vi "All Not Complex.vi"() -> (3 "Benchmark":cluster{i32[], dbl[]}[](graph))   [LabVIEW 2020]
doc: "Execute GEMM Process for different size on different Toolkits (Accelerator/Culab/CUDA/LabVIEW/G2CPU) and LabVIEW(CPU)."
uses:
  Source/_Controls/acc_execution_provider_enum.ctl
panel:
  out "Accelerator CUDA":bool
  out "Culab":bool
  out "Accelerator TRT":bool
  out "LabVIEW":bool
  out "G2CPU":bool
  out "LabVIEW Toolkit Time":dbl
  out "G2CPU Time":dbl
  out "Accelerator CUDA Times":dbl[](array[numeric])
  out "Accelerator CUDA Time":dbl
  out "LabVIEW Times":dbl[](array[numeric])
  out "G2CPU Times":dbl[](array[numeric])
  out "Culab Times":dbl[](array[numeric])
  out "Accelerator TRT Times":dbl[](array[numeric])
  out "Culab Time":dbl
  out "Accelerator TRT Time":dbl
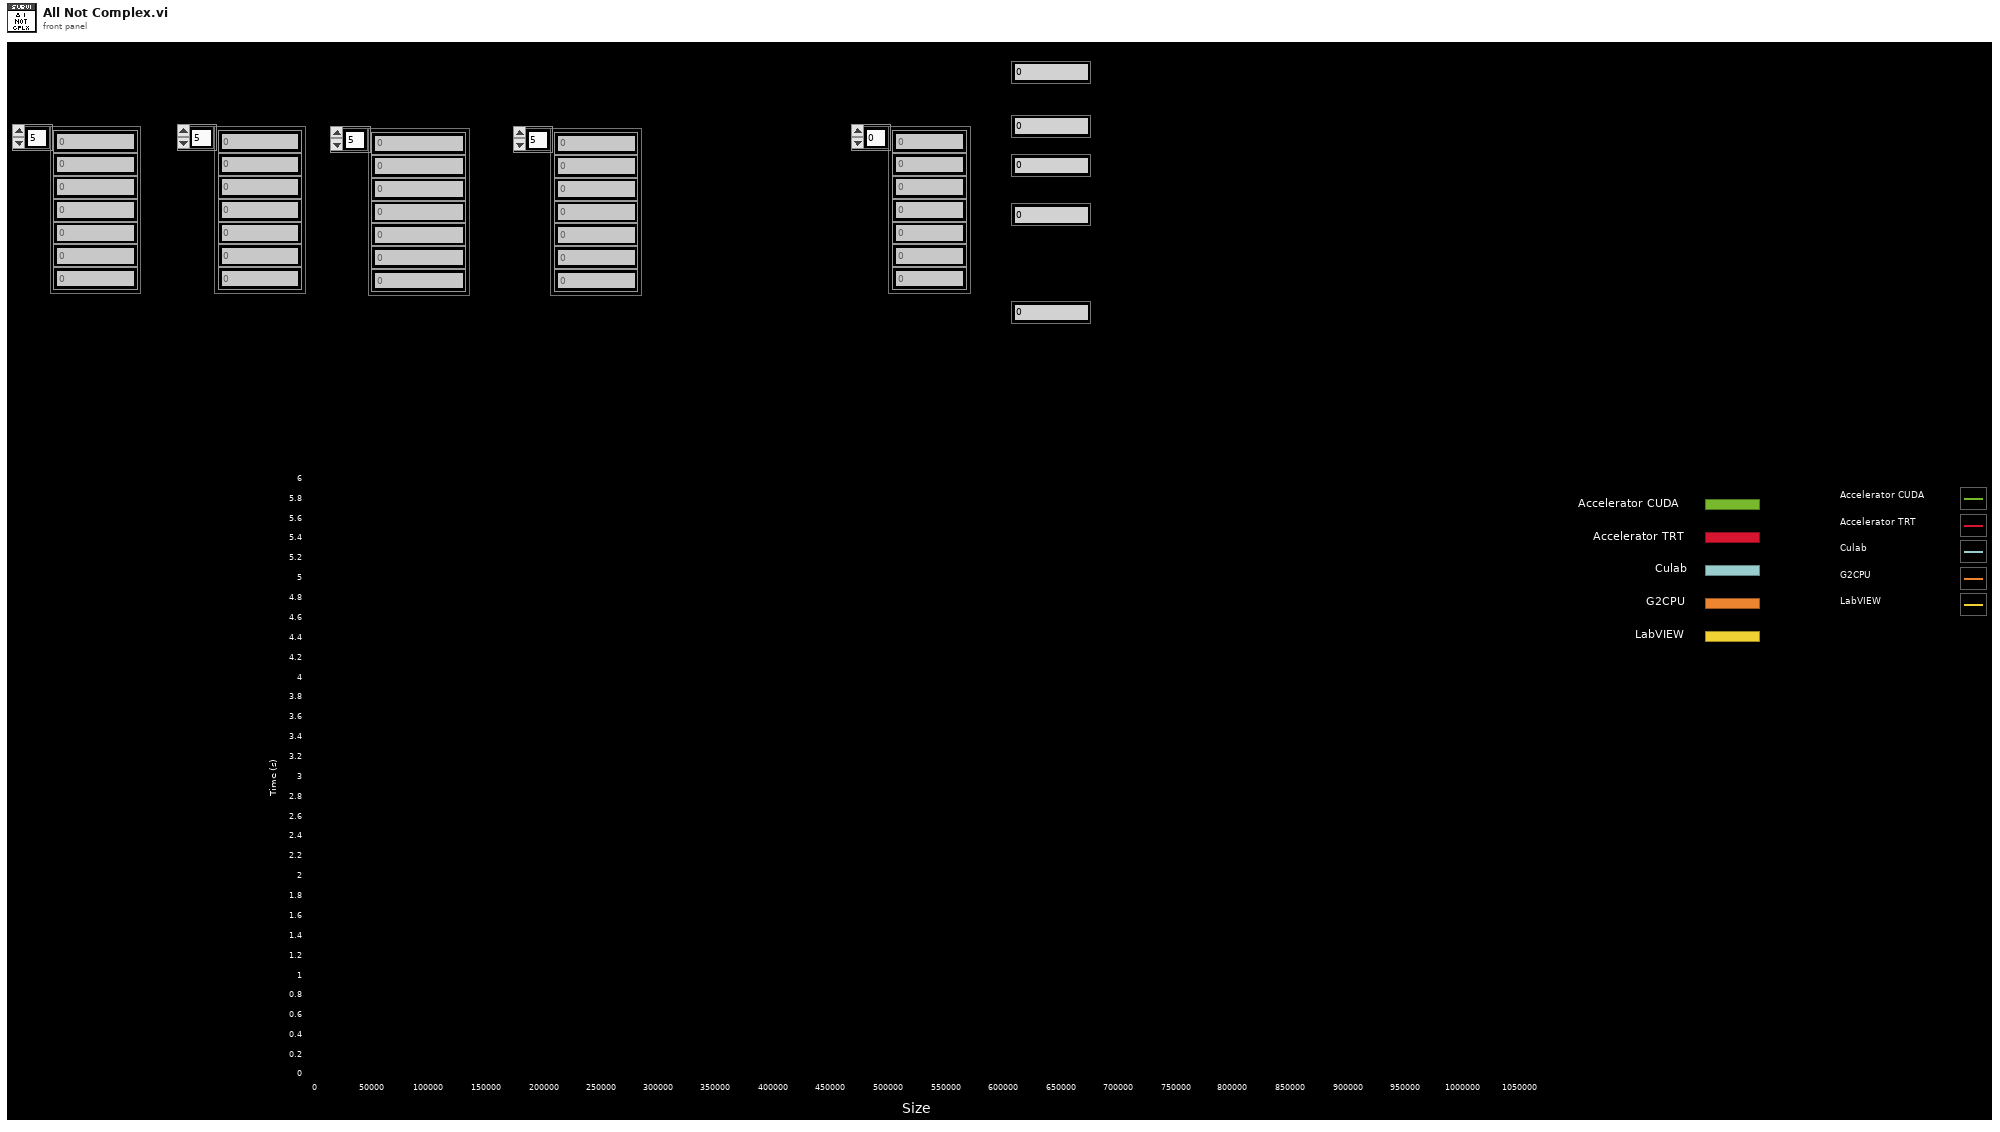
[diagram p1: front panel]
types:
  T1 = cluster{"intra_op_num_threads":i32, "inter_op_num_threads":i32, "execution_mode":enum16{"ORT_SEQUENTIAL", "ORT_PARALLEL"}, "deterministic_compute":bool, "graph_optimization_level":u16, "optimized_model_file_path":path, "profiling output dir":path}
  T2 = typedef "acc_execution_provider_enum.ctl" = enum16{"CPU", "CUDA", "TensorRT"}
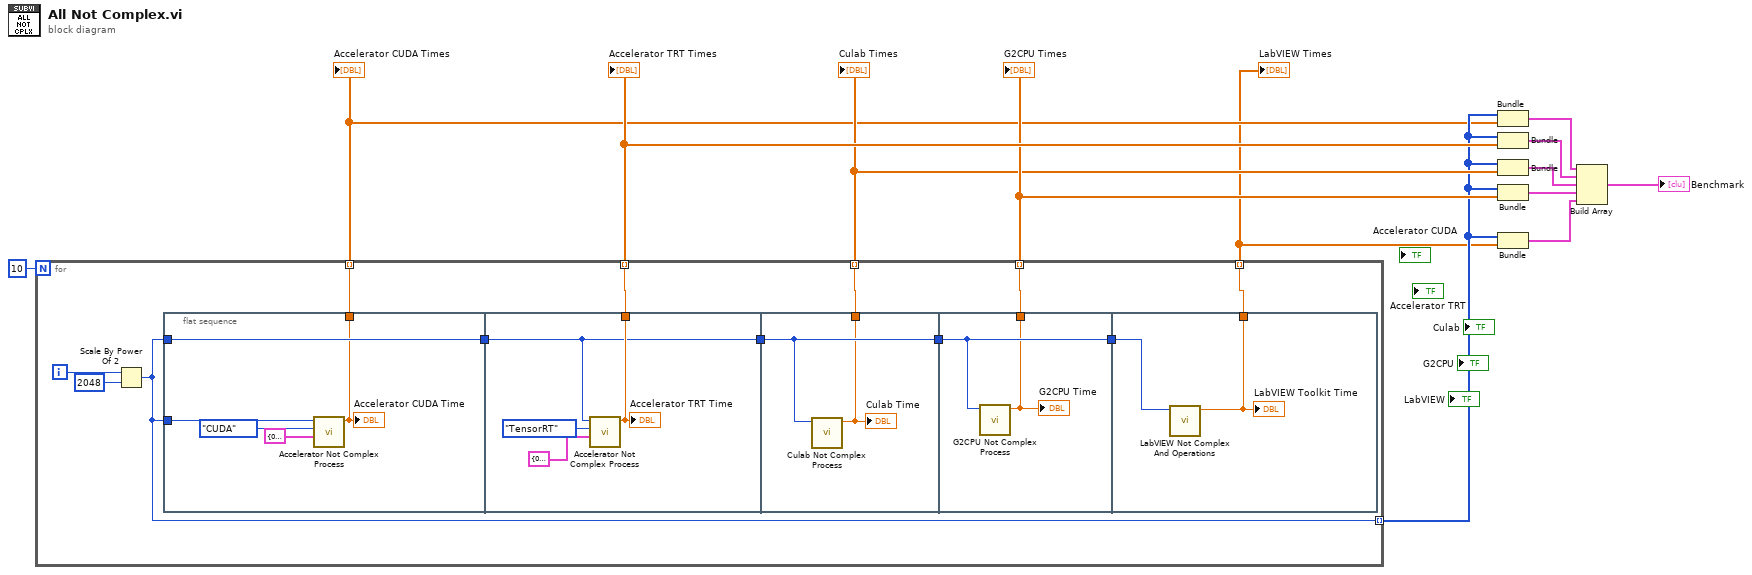
[diagram p0: block diagram]
diagram:
  n1 = for {
    N: 10 -> [_]
    tunnel: [w23] -> w12 mode=indexing
    tunnel: [w22] -> w10 mode=indexing
    tunnel: [w21] -> w11 mode=indexing
    tunnel: [w17] -> w4 mode=indexing
    tunnel: [w15] -> w3 mode=indexing
    tunnel: [w14] -> w2 mode=indexing
    i -> [w19]
    n2 = Scale By Power Of 2(n=w19, x=2048) -> (x*2^n=w17:i32)
    n3 = flat-sequence {
      tunnel: w17 -> [w30]
      tunnel: w17 -> [w28]
      tunnel: [w30] -> w16
      tunnel: [w27] -> w15
      tunnel: [w33] -> w25
      tunnel: [w34] -> w23
      tunnel: w16 -> [w33]
      tunnel: w25 -> [w36]
      tunnel: [w36] -> w24
      tunnel: [w35] -> w22
      tunnel: w24 -> [w38]
      tunnel: [w37] -> w21
      tunnel: [w38] -> w18
      tunnel: [w39] -> w14
      tunnel: w18 -> [w40]
      frame #0 {
        n4 = call "Accelerator Not Complex Process.vi"("Sessions Parameters"=T1 {"intra_op_num_threads"=0, "inter_op_num_threads"=0, "execution_mode"=enum."ORT_SEQUENTIAL", "deterministic_compute"=FALSE, "graph_optimization_level"=1, "optimized_model_file_path"=path "", "profiling output dir"=path ""}, "Execution Device"=acc_execution_provider_enum."CUDA", "X size"=w28) -> ("Accelerator Time"=w27:dbl)  [unwired: 8 in]
        "Accelerator CUDA Time" <- w27
      }
      frame #1 {
        n5 = call "Accelerator Not Complex Process.vi"("Sessions Parameters"=T1 {"intra_op_num_threads"=0, "inter_op_num_threads"=0, "execution_mode"=enum."ORT_SEQUENTIAL", "deterministic_compute"=FALSE, "graph_optimization_level"=1, "optimized_model_file_path"=path "", "profiling output dir"=path ""}, "Execution Device"=acc_execution_provider_enum."TensorRT", "X size"=w33) -> ("Accelerator Time"=w34:dbl)  [unwired: 8 in]
        "Accelerator TRT Time" <- w34
      }
      frame #2 {
        n6 = call "Culab Not Complex Process.vi"("X size"=w36) -> ("Culab Time"=w35:dbl)  [unwired: 10 in]
        "Culab Time" <- w35
      }
      frame #3 {
        n7 = call "G2CPU Not Complex Process.vi"("X size"=w38) -> ("G2CPU Time"=w37:dbl)  [unwired: 10 in]
        "G2CPU Time" <- w37
      }
      frame #4 {
        n8 = call "LabVIEW Not Complex And Operations.vi"("X size"=w40) -> ("LabVIEW Time"=w39:dbl)  [unwired: 10 in]
        "LabVIEW Toolkit Time" <- w39
      }
    }
  }
  "Accelerator TRT Times" <- w12
  "Culab Times" <- w10
  "G2CPU Times" <- w11
  "LabVIEW Times" <- w2
  "Accelerator CUDA Times" <- w3
  n9 = Bundle(w4, w3) -> (w5:cluster{i32[], dbl[]})  [unwired: 1 in]
  n10 = Bundle(w4, w12) -> (w6:cluster{i32[], dbl[]})  [unwired: 1 in]
  n11 = Bundle(w4, w10) -> (w9:cluster{i32[], dbl[]})  [unwired: 1 in]
  n12 = Bundle(w4, w11) -> (w8:cluster{i32[], dbl[]})  [unwired: 1 in]
  n13 = Bundle(w4, w2) -> (w1:cluster{i32[], dbl[]})  [unwired: 1 in]
  n14 = Build Array(w5, w6, w9, w8, w1) -> (→"Benchmark":cluster{i32[], dbl[]}[])
